vi "Get SMO Public API.vi"(8 "error in (no error)":errorcluster, 11 "Instrument.sample-registry":refnum<class "Instrument.sample-registry.lvclass">) -> (0 "error out":errorcluster, 2 "Commands":string[](array[string]), 3 "Instrument.sample-registry out":refnum<class "Instrument.sample-registry.lvclass">)   [LabVIEW 2019, in "Instrument.sample-registry.lvclass"]
uses:
  Instrument.sample-registry.lvclass
  Typedefs/Instrument.sample-registry.Commands--Enum.ctl
  94fc51da-4a6c-4076-b8e5-59f202131845.vi
  <userlib>/LevyLab/Levylab Instruments/Instrument Types/VSource/Instrument.VSource.lvclass
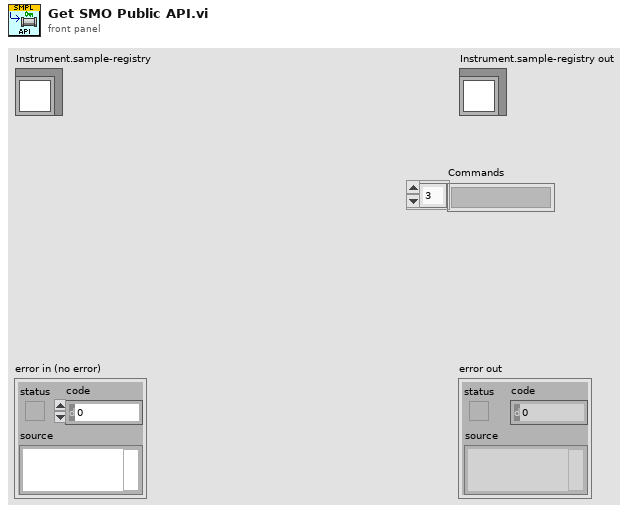
[diagram p1: front panel]
types:
  T1 = typedef "Instrument.sample-registry.lvclass/Instrument.sample-registry.Commands--Enum.ctl" = enum16{"Set User", "Get User", "Set Sample", "Get Sample"}
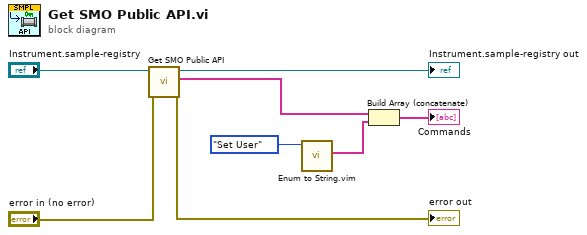
[diagram p0: block diagram]
diagram:
  n1 = call-parent "Get SMO Public API.vi"("error in (no error)"="error in (no error)", "Instrument in"="Instrument.sample-registry") -> ("error out"=→"error out":errorcluster, "Commands"=w8:string[], "Instrument out"=→"Instrument.sample-registry out":refnum<class "Instrument.sample-registry.lvclass">)  [unwired: 7 in]
  n2 = call "Enum to String.vim"("Command"=Instrument.sample-registry.Commands--Enum."Set User" ("Commands")) -> ("Commands []"=w3:string[])  [unwired: 9 in, 1 out]
  n3 = Build Array (concatenate)(w8, w3) -> (→"Commands":string[])
